vi "Replace Image.vi"(8 "error in":errorcluster, 9 "image item":i32, 10 "PNG Image File":path, 11 "LabVIEW File with Button":path) -> (0 "error out":errorcluster, 3 "File with Button (dup)":path)   [LabVIEW 2026, in "TSC Material Theme.lvlib" / "Material-Scheme.lvclass"]
doc: "This example VI was obtained from this post: \n\nhttps://forums.ni.com/t5/LabVIEW-APIs-Discussions/Set-TRUE-FALSE-Image-of-a-boolean-control-automatically-using/m-p/3419083/highlight/true#M868\n\n<b>WARNING</b>\nThis VI uses a dll call to the resource file for a LabVIEW VI/CTL - it is searching the binary data for the PNG images that the VI or CTL contains\n\n<b>Code Developed By:</b> +\nDaniel Coons +\nTechnology Service Corporation +\nwww.tsc.com/atcs"
uses:
  Material-Scheme.lvclass
panel:
  out "Resources":string[](array[string])
  # "For DEBUG"
  # "MNGI resources are 6 images\non buttons (pressed, hover, etc)"
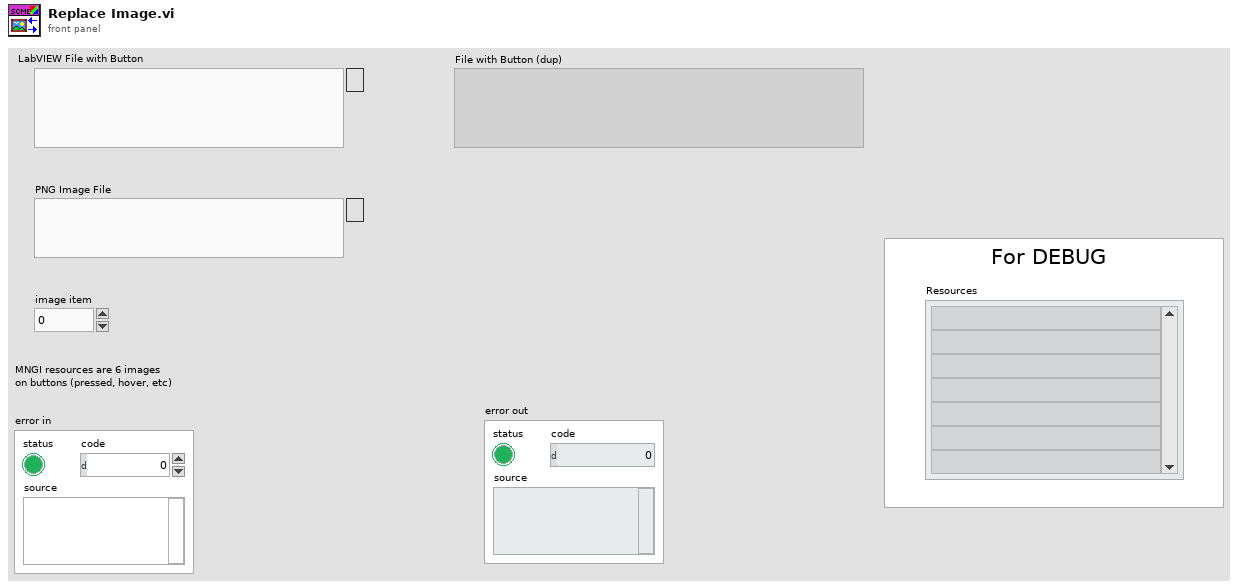
[diagram p1: front panel]
types:
  T1 = cluster{"type":u32, "id":i32, "name":string, "binary data":string}[]
  T2 = cluster{"type":u32, "id":i32, "name":string, "binary data":string}
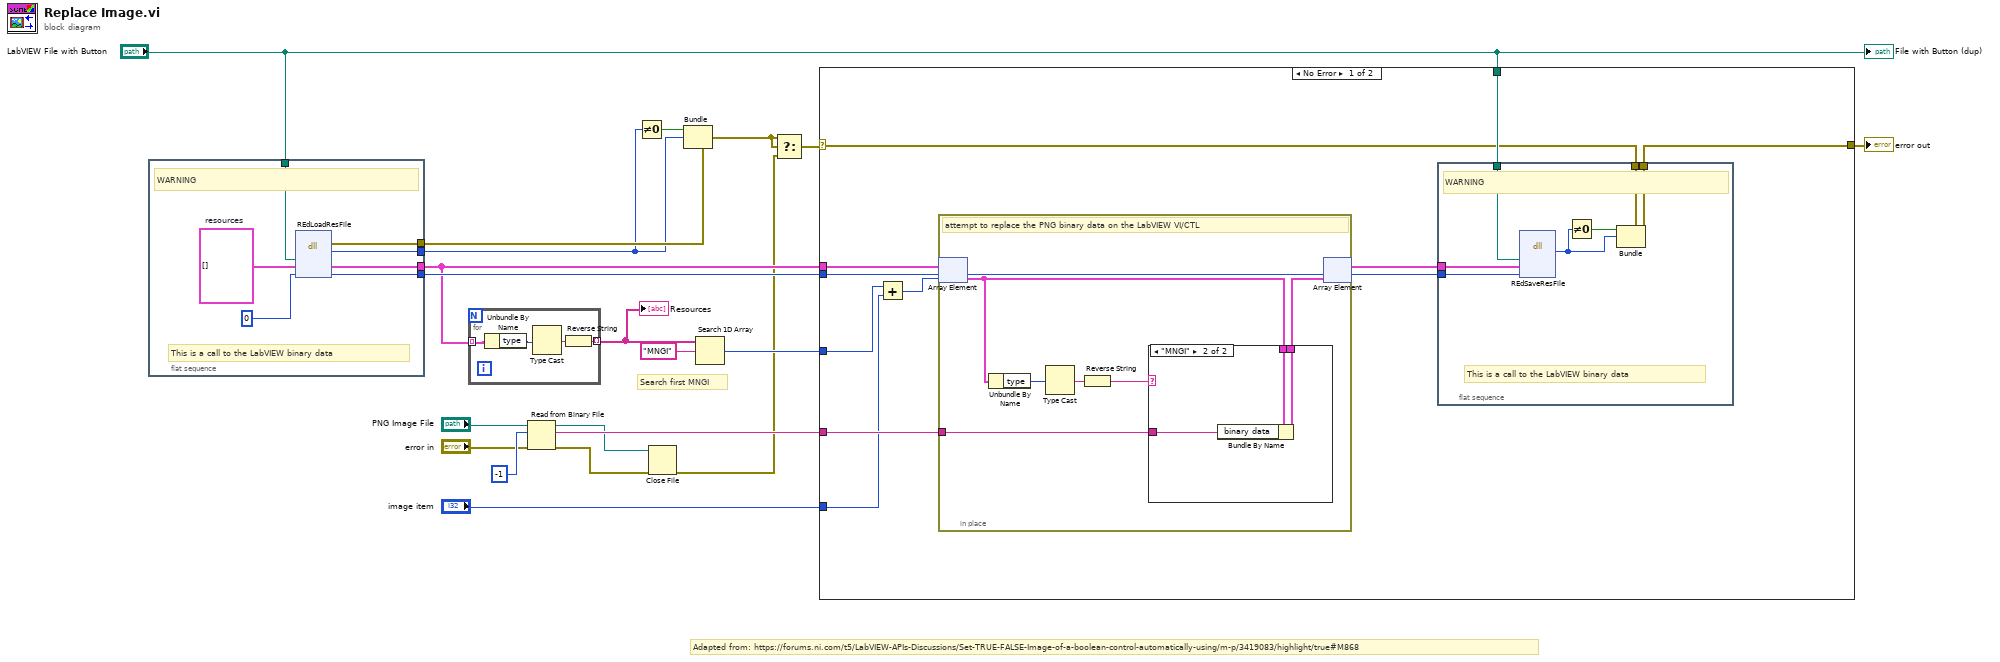
[diagram p0: block diagram]
diagram:
  # "Adapted from: https://forums.ni.com/t5/LabVIEW-APIs-Discussions/Set-TRUE-FALSE-Image-of-a-boolean-control-automatically-using/m-p/3419083/highlight/true#M868"
  # "Search first MNGI"
  n1 = flat-sequence {
    tunnel: [w25] -> w20
    tunnel: [w24] -> w18
    tunnel: [w23] -> w17
    tunnel: [w22] -> w16
    tunnel: "LabVIEW File with Button" -> [w21]
    frame #0 {
      w27 = T1 []  # resources
      # "This is a call to the LabVIEW binary data"
      # "WARNING"
      n2 = dll-call lib="LabVIEW" fn="REdLoadResFile"("path"=w21, "resources"=w27, "type"=0) -> (error out=w25:errorcluster, "return type"=w24:i32, "resources"=w22:T1, "type"=w23:i32)  [unwired: 3 in, 2 out]
    }
  }
  n3 = for {
    tunnel: w16 -> [w31] mode=indexing
    tunnel: [w28] -> w3 mode=indexing
    n4 = Unbundle By Name(w31) -> ("type"=w29:u32)
    n5 = Type Cast(x=w29) -> (*(type *) &x=w30:string)  [unwired: 1 out]
    n6 = Reverse String(1:w30) -> (0:w28:string)
  }
  "Resources" <- w3
  n7 = Read from Binary File(8:"error in", 10:-1 ("count"), 11:"PNG Image File") -> (0:w8:errorcluster, 2:w11:string, 3:w4:refnum<file>)  [unwired: 4 out]
  n8 = Not Equal To 0?(x=w18) -> (x != 0?=w19:bool)
  n9 = Close File(refnum=w4, error in=w8) -> (error out=w5:errorcluster)  [unwired: 1 out]
  n10 = Bundle(cluster=w20, "status"=w19, "code"=w18) -> (w10:errorcluster)  [unwired: 1 out]
  n11 = Search 1D Array(1D array=w3, element="MNGI") -> (index of element=w14:i32)  [unwired: 1 out]
  n12 = Select(t=w10, s=w10, f=w5) -> (s? t:f=w9:errorcluster)
  n13 = case shown="No Error" w9 {
    selector: w9 -> [w37 w59]
    tunnel: [w34 w59] -> w1
    tunnel: "LabVIEW File with Button" -> [w40 _]
    tunnel: w16 -> [w41 _]
    tunnel: w17 -> [w38 _]
    tunnel: w14 -> [w36 _]
    tunnel: w11 -> [w35 _]
    tunnel: "image item" -> [w32 _]
    frame No Error {
      n14 = Add(x=w36, y=w32) -> (x+y=w33:i32)
      n15 = in-place {
        in-place-border: w35 -> [w54]
        # "attempt to replace the PNG binary data on the LabVIEW VI/CTL"
        n16 = in-place-array #1(w41, w33) -> (w52:T2)
        n17 = Unbundle By Name(w52) -> ("type"=w50:u32)
        n18 = Type Cast(x=w50) -> (*(type *) &x=w51:string)  [unwired: 1 out]
        n19 = Reverse String(1:w51) -> (0:w49:string)
        n20 = case shown="\"MNGI\"" w49 {
          tunnel: w54 -> [_ w56]
          tunnel: [w55 w58] -> w53
          tunnel: w52 -> [w55 w57]
          frame Default {
          }
          frame "MNGI" {
            n21 = Bundle By Name(cluster=w57, "binary data"=w56) -> (w58:T2)
          }
        }
        n22 = in-place-array #1(w53) -> (w39:T1)  [unwired: 1 out]
      }
      n23 = flat-sequence {
        tunnel: w40 -> [w48]
        tunnel: w39 -> [w47]
        tunnel: w38 -> [w46]
        tunnel: w37 -> [w45]
        tunnel: [w44] -> w34
        frame #0 {
          # "This is a call to the LabVIEW binary data"
          # "WARNING"
          n24 = dll-call lib="LabVIEW" fn="REdSaveResFile"("path"=w48, "resources"=w47, "type"=w46) -> ("return type"=w42:i32)  [unwired: 6 in, 2 out]
          n25 = Not Equal To 0?(x=w42) -> (x != 0?=w43:bool)
          n26 = Bundle(cluster=w45, "status"=w43, "code"=w42) -> (w44:errorcluster)  [unwired: 1 out]
        }
      }
    }
    frame Error {
    }
  }
  "error out" <- w1
  "File with Button (dup)" <- "LabVIEW File with Button"
